vi "ScaledWaveform-RemoveResultWaveforms.vi"(8 "Error in":errorcluster, 11 "Custom Device ref":T1 format="%.0x") -> (0 "Error out":errorcluster, 3 "Custom Device ref out":T1 format="%.0x")   [LabVIEW 2023, in "Waveform-Processing-Custom-Device Shared.lvlib" / "Scaled Waveform.lvlib"]
uses:
  Scaled Waveform.lvlib
  <vilib>/NI VeriStand/Custom Device API/Custom Device Item Ref.ctl
  Constants.vi
  <vilib>/NI VeriStand/Custom Device API/Get Item Property (Dependent Node Pointer).vi
  System Explorer/Waveform-Processing-Custom-Device System Explorer.lvlib
  <vilib>/NI VeriStand/Custom Device API/Custom Device API.lvlib
  Waveform-Processing-Custom-Device Shared.lvlib
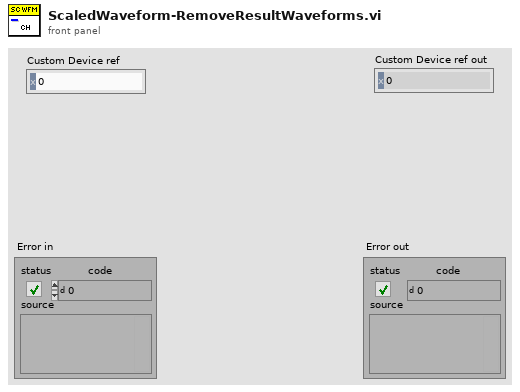
[diagram p1: front panel]
types:
  T1 = typedef "Custom Device API.lvlib/Custom Device Item Ref.ctl" = u64
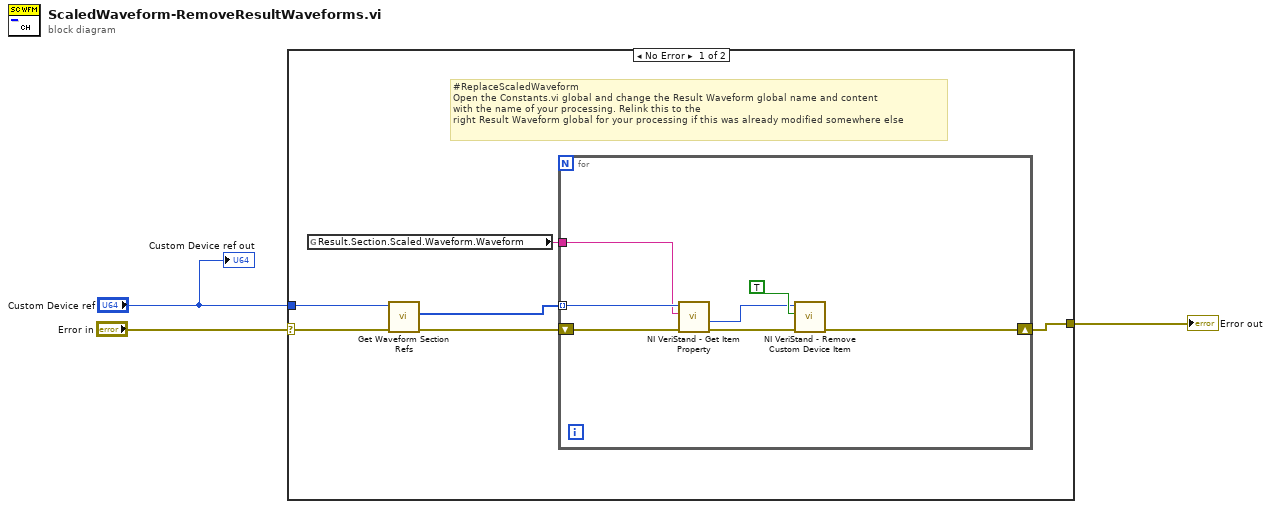
[diagram p0: block diagram]
diagram:
  n1 = case shown="No Error" "Error in" {
    selector: "Error in" -> [w9 w17]
    tunnel: "Custom Device ref" -> [w8 _]
    tunnel: [w5 w17] -> w2
    frame No Error {
      # "#ReplaceScaledWaveform \nOpen the Constants.vi global and change the Result Waveform global name and content \nwith the name of your processing. Relink this to the \nright Result Waveform global for your processing if this was already modified somewhere else"
      n2 = global read "Constants.vi" "Result.Section.Scaled.Waveform.Waveform"() -> (w4:string)
      n3 = call "Get Waveform Section Refs.vi"("Error in"=w9, "Device Ref in"=w8) -> ("Error out"=w7:errorcluster, "Result Section Refs"=w6:T1[])  [unwired: 7 in, 1 out]
      n4 = for {
        tunnel: w6 -> [w15] mode=indexing
        shift-right: [w10] -> w5
        shift-left: w7 -> [w16]
        tunnel: w4 -> [w12]
        n5 = call-poly <vilib>:"NI VeriStand - Get Item Property.vi"("error in (no error)"=w16, "Property Name"=w12, "Item Ref in"=w15) -> ("error out"=w13:errorcluster, "Dependent Node Ref"=w11:T1)  [unwired: 5 in, 2 out]
        n6 = call <vilib>:"NI VeriStand - Remove Custom Device Item.vi"("error in (no error)"=w13, "Force Delete (F)"=TRUE, "Item Ref in"=w11) -> ("error out"=w10:errorcluster)  [unwired: 7 in, 1 out]
      }
    }
    frame Error {
    }
  }
  "Error out" <- w2
  "Custom Device ref out" <- "Custom Device ref"
